vi "SRV_Write Sensors Config File.vi"(0 "Sensors Config File Path":path, 7 "Sensors Config":T1[](array[typedef]) {"Register" format="%.0x"; "I2C Address" format="%.0x"; "Sample Period (ms)" min=10 max=60000 step=1; "Digital Mask" format="%.0x"; "Channel" format="%.0x"}, 11 "error in (no error)":errorcluster) -> (15 "error out":errorcluster)   [LabVIEW 2009]
uses:
  SRV_Sensor Config Cluster.ctl
  SRV_Sensor Analog-Digital.ctl
  SRV_Sensor Sampling Mode.ctl
  SRV_Sensor View Config Cluster.ctl
  SRV_Sensors Names.ctl
  SRV_Sensor PicoC Shared Var Type.ctl
  <vilib>/Utility/xml.llb/Write to XML File(string).vi
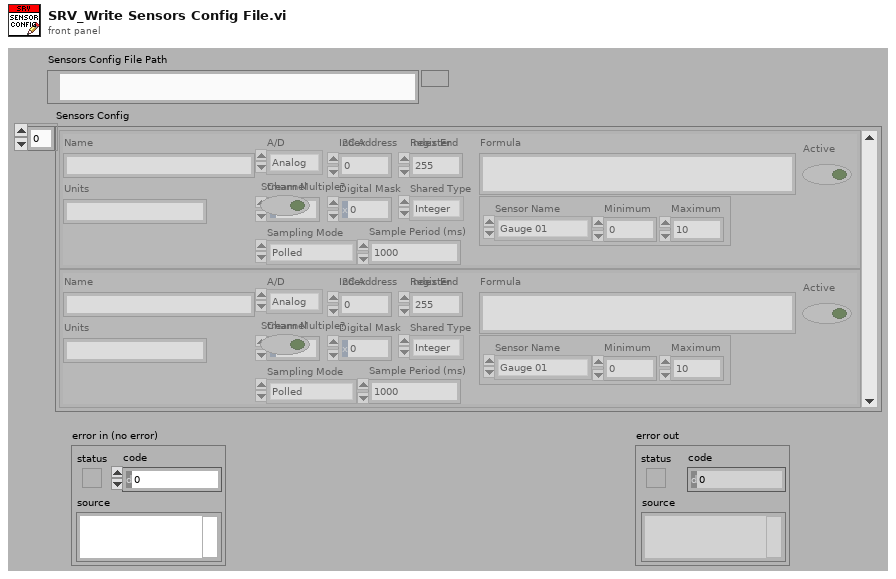
[diagram p1: front panel]
types:
  T1 = typedef "SRV_Sensor Config Cluster.ctl" = cluster{"Name":string, "A/D":T2, "I2C Address":u8, "Register":u8, "Channel":u8, "Digital Mask":u8, "Units":string, "Sampling Mode":T3, "Sample Period (ms)":u32, "Formula":string, "Sensor View Config":T4, "Active":bool, "PicoC Shared Var Type":T6, "Index":u8, "Stream Multiple?":bool, "Index End":u8}
  T2 = typedef "SRV_Sensor Analog-Digital.ctl" = enum16{"Analog", "Digital", "RCMx1 Analog", "PicoC Shared"}
  T3 = typedef "SRV_Sensor Sampling Mode.ctl" = enum16{"Polled", "Streaming"}
  T4 = typedef "SRV_Sensor View Config Cluster.ctl" = cluster{"Sensor Name":T5, "Minimum":dbl, "Maximum":dbl}
  T5 = typedef "SRV_Sensors Names.ctl" = enum16{"Gauge 01", "Gauge 02", "Gauge 03", "Gauge 04", "Meter 01", "Meter 02", "Meter 03", "Meter 04", "Numeric 01", "Numeric 02", "Numeric 03", "Numeric 04", "Numeric 05", "Numeric 06", "Numeric 07", "Numeric 08", "Boolean 01", "Boolean 02", "Boolean 03", "Boolean 04", "Boolean 05", "Boolean 06", "Boolean 07", "Boolean 08", "Boolean 09", "Boolean 10", "Boolean 11", "Boolean 12", "Boolean 13", "Boolean 14", "Boolean 15", "Boolean 16", "Boolean 17", "Boolean 18", "Boolean 19", "Boolean 20", "Boolean 21", "Boolean 22", "Boolean 23", "Boolean 24", "Boolean 25", "Boolean 26", "Boolean 27", "Boolean 28", "Boolean 29", "Boolean 30", "Boolean 31", "Boolean 32"}
  T6 = typedef "SRV_Sensor PicoC Shared Var Type.ctl" = enum16{"String", "Integer", "Float"}
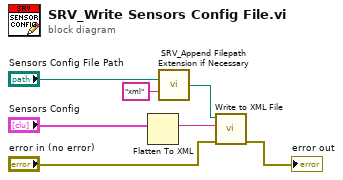
[diagram p0: block diagram]
diagram:
  n1 = Flatten To XML(anything="Sensors Config") -> (xml string=w6:string)
  n2 = call "SRV_Append Filepath Extension if Necessary.vi"("Filepath"="Sensors Config File Path", "Extension"="xml") -> ("Filepath with Extension"=w4:path)  [unwired: 13 in]
  n3 = call-poly <vilib>:"Write to XML File.vi"("error in (no error)"="error in (no error)", "XML Input"=w6, "XML File Path"=w4) -> ("error out"=→"error out":errorcluster)  [unwired: 6 in, 2 out]
